vi "DAQmx Create Channel (CI-Duty Cycle).vi"(0 "task in":refnum<k21>, 1 "maximum frequency":dbl=10000.0 format="%0.6f", 2 "minimum frequency":dbl=2.0 format="%0.6f", 5 "counter":tag, 7 "name to assign":string, 11 "error in":errorcluster, 12 "custom scale name":tag, 13 "starting edge":i32(ring)=10280 items=["Rising"=10280, "Falling"=10171]) -> (4 "task out":refnum<k21>, 15 "error out":errorcluster)   [LabVIEW 2013]
doc: "Creates channel(s) to duty cycle of a digital pulse. Connect the input signal to the default input terminal of the counter unless you select a different input terminal. With the exception of devices that support multi-counter tasks, you can create only one counter input channel at a time with this VI because a task can contain only one counter input channel. To read from multiple counters simultaneously, use a separate task for each counter."
uses:
  <resource>/objmgr/daqmx.rc
panel:
  # "input limits"
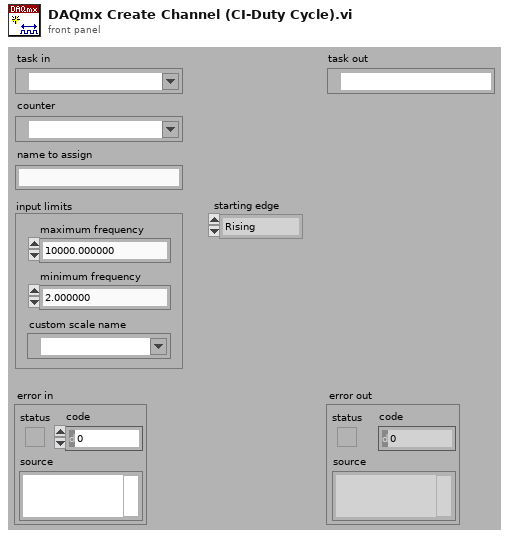
[diagram p1: front panel]
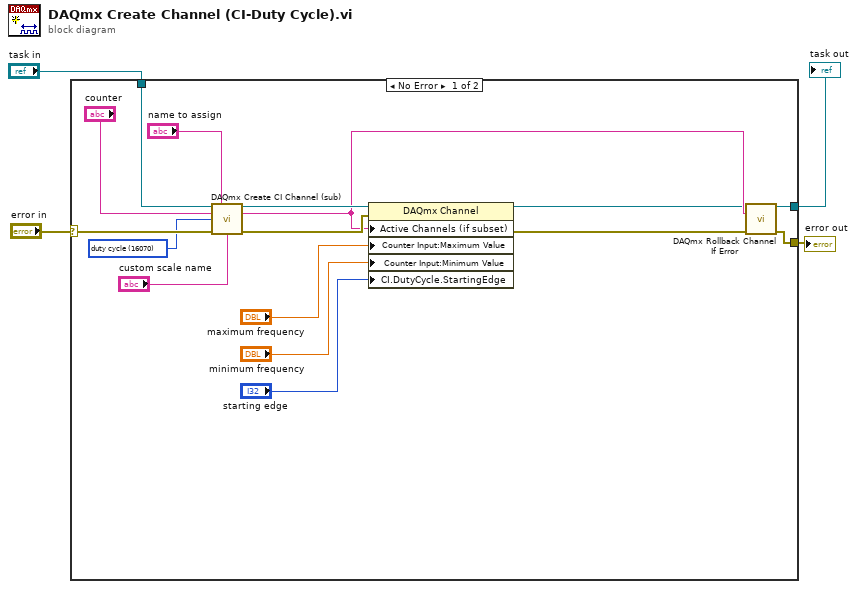
[diagram p0: block diagram]
diagram:
  n1 = case shown="No Error" "error in" {
    selector: "error in" -> [w19 w21]
    tunnel: "task in" -> [w20 w22]
    tunnel: [w9 w22] -> w2
    tunnel: [w8 w21] -> w1
    frame No Error {
      w13 = 16070 items=["count events"=10125, "frequency"=10179, "period"=10256, "pulse width"=10267, "semi period"=10289, "duty cycle"=16070] ("measurement type")
      n2 = call "DAQmx Create CI Channel (sub).vi"("task in"=w20, "virtual channel name"="name to assign", "physical channel name"="counter", "measurement type"=w13, "error in"=w19, "custom scale"="custom scale name") -> ("task out"=w10:refnum<k21>, "channel names"=w7:string, "error out"=w17:errorcluster)  [unwired: 7 out]
      n3 = property class="DAQmx Channel"(reference=w10, error in=w17, "Active Channels (if subset)"=w7, "Counter Input:Maximum Value"="maximum frequency", "Counter Input:Minimum Value"="minimum frequency", "CI.DutyCycle.StartingEdge"="starting edge") -> (reference out=w5:refnum<k21>, error out=w6:errorcluster)
      n4 = call "DAQmx Rollback Channel If Error.vi"("task in"=w5, "channel names"=w7, "error in"=w6) -> ("task out"=w9:refnum<k21>, "error out"=w8:errorcluster)  [unwired: 11 out]
    }
    frame Error {
    }
  }
  "error out" <- w1
  "task out" <- w2
